vi "Teff_Calc_Recurring.vi"(8 "eTRF In":dbl, 9 "Length In":dbl, 10 "Bed Temp":dbl, 11 "TRF":dbl) -> (0 "eTRF Out":dbl, 1 "Length Out":dbl, 2 "Teff":dbl)   [LabVIEW 2014]
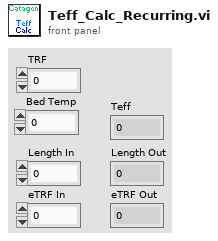
[diagram p1: front panel]
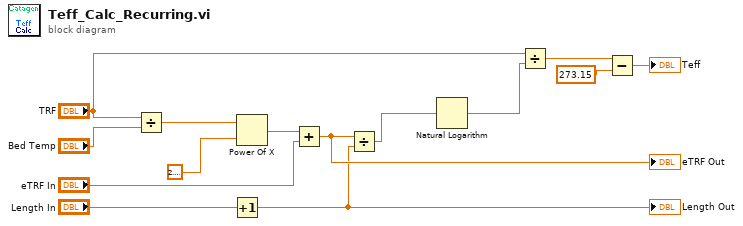
[diagram p0: block diagram]
diagram:
  n1 = Divide(x="TRF", y="Bed Temp") -> (x/y=w13:dbl)
  n2 = Increment(x="Length In") -> (x+1=w1:dbl)
  "Length Out" <- w1
  n3 = Power Of X(1:2.718281828459045, 2:w13) -> (0:w5:dbl)
  n4 = Add(x=w5, y="eTRF In") -> (x+y=w3:dbl)
  "eTRF Out" <- w3
  n5 = Divide(x=w3, y=w1) -> (x/y=w11:dbl)
  n6 = Natural Logarithm(1:w11) -> (0:w10:dbl)
  n7 = Divide(x="TRF", y=w10) -> (x/y=w7:dbl)
  n8 = Subtract(x=w7, y=273.15) -> (x-y=→"Teff":dbl)
